vi "Configure Scaling.vi"(8 "error in (no error)":errorcluster, 9 "Current Sacling (1.0000)":dbl=1.0 caption="Current Scaling (1.0000)" min=1e-06 max=1000000.0 step=1.0 format="%.6f", 10 "Voltage Sacling (1.0000)":dbl=1.0 caption="Voltage Scaling (1.0000)" min=1e-06 max=1000000.0 step=1.0 format="%.6f", 11 "VISA resource name":refnum<visa-resource-name>) -> (0 "error out":errorcluster, 3 "VISA resource name out":refnum<visa-resource-name>)   [LabVIEW 2015, in "Voltech PM1000+.lvlib"]
doc: "Configures both voltage and current scaling factors. It also indicates the voltage and current scaling factors.\n\nA current transformer produces an output current which is proportional to the load current being measured. For example, the Voltech CL100 produces an output current that is 1/100 of the current being measured.\n\nTo measure the correct current on the PM1000+, use the scale function of the analyzer to scale, or multiply, the CT output current.\n\nFor example, the CL100 is a 100:1 CT. When measuring 100A, its output is 1A. To scale this on the PM1000+, a scale factor of 100 must be entered. And PM1000+ is now ready to make measurements using a CT."
uses:
  <instrlib>/Voltech PM1000+/Voltech PM1000+.lvlib
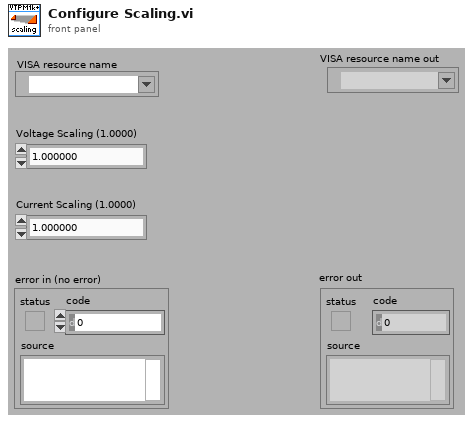
[diagram p1: front panel]
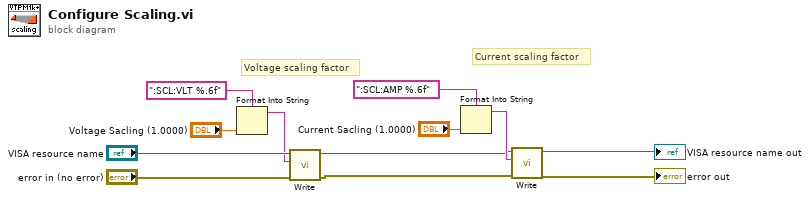
[diagram p0: block diagram]
diagram:
  # "Current scaling factor"
  # "Voltage scaling factor"
  n1 = Format Into String(format string=":SCL:VLT %.6f", "Voltage Sacling (1.0000)") -> (resulting string=w6:string)  [unwired: 2 in, 1 out]
  n2 = call <instrlib>:"Write.vi"("error in (no error)"="error in (no error)", "Write Buffer"=w6, "VISA resource name"="VISA resource name") -> ("error out"=w3:errorcluster, "VISA resource name out"=w4:refnum<visa-resource-name>)  [unwired: 7 in]
  n3 = Format Into String(format string=":SCL:AMP %.6f", "Current Sacling (1.0000)") -> (resulting string=w5:string)  [unwired: 2 in, 1 out]
  n4 = call <instrlib>:"Write.vi"("error in (no error)"=w3, "Write Buffer"=w5, "VISA resource name"=w4) -> ("error out"=→"error out":errorcluster, "VISA resource name out"=→"VISA resource name out":refnum<visa-resource-name>)  [unwired: 7 in]
